vi "application.vi"() -> ()   [LabVIEW 2017, in "application.lvlib" / "application.lvclass"]
uses:
  application.lvclass
  application.lvclass/application.ctl
  <userlib>/NEVSTOP-Programming-Palette/Dialog & Interface/Fit VI window to Content_nevstop.vi
  <vilib>/Utility/config.llb/NI_LVConfig.lvlib
  <userlib>/NEVSTOP-Programming-Palette/Configuration/_OpenG Variant Configuration File/OpenG Variant Configuration File_nevstop.lvlib
panel:
  in  "Tab Control":enum32{"Main", "Settings"}(tab)
  out "version detected":string caption="File Path"
  in  "Settings":bool
  out "CMD":string caption="CMD Line"
  in  "file path":path=path "D:/Projects/Personal/Multi-LabVIEW-Selector/Multi-LabVIEW Selector.lvproj" caption="File Path"
  in  "LabVIEW List":string(combo)
  in  "OK":bool
  in  "Cancel":bool
  in  "Display Time(ms)":i32 min=0 max=10000 step=100
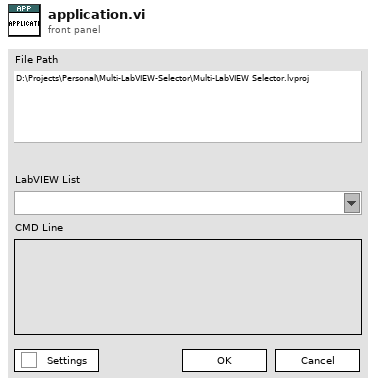
[diagram p1: front panel]
types:
  T1 = enum32{"invalid app kind", "Development System", "Run Time System", "Student Edition", "Embedded LabVIEW", "Evaluation", "Custom"}
  T2 = enum32{"Invalid", "Standard", "Closed", "Hidden", "Minimized", "Maximized"}
  T3 = cluster{"Core":cluster{"Current VI Reference":refnum<vi>, "Close Panel on Exit?":bool}, "RuntimeEngine":bool, "ConfigFilePath":path}
  T4 = cluster{"Current VI Reference":refnum<vi>, "Close Panel on Exit?":bool}
  T5 = typedef "NI_LVConfig.lvlib/Config Data RefNum.ctl" = refnum<k1>
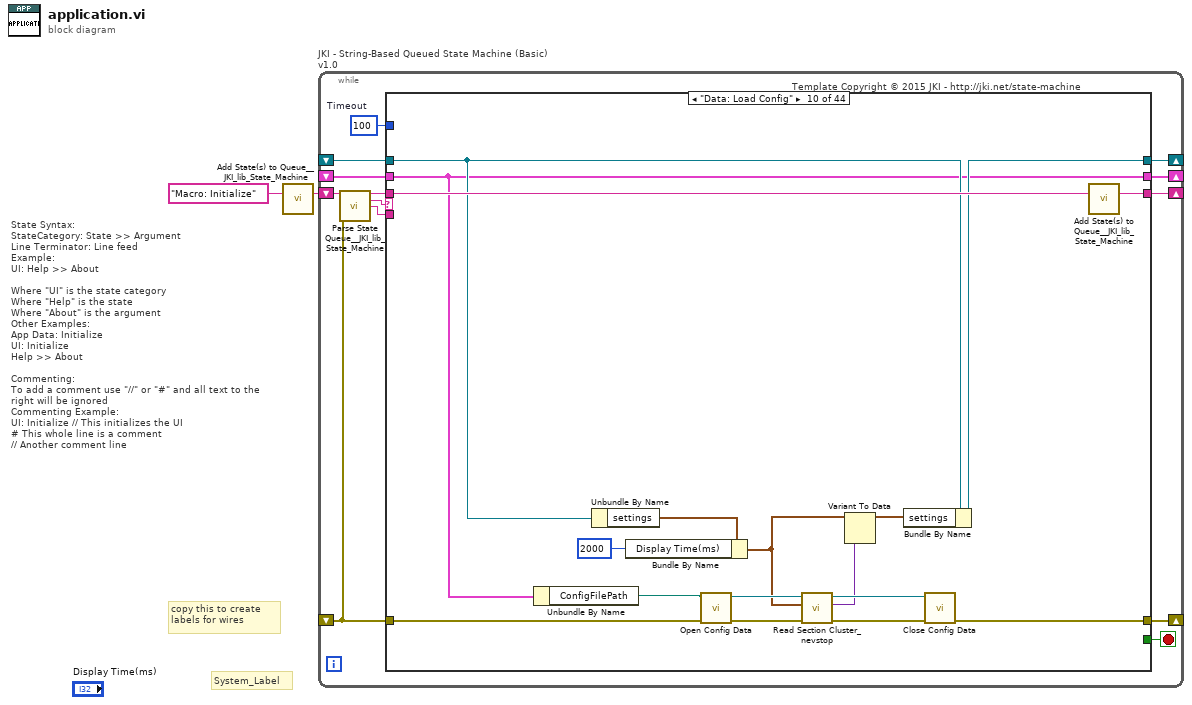
[diagram p0: block diagram]
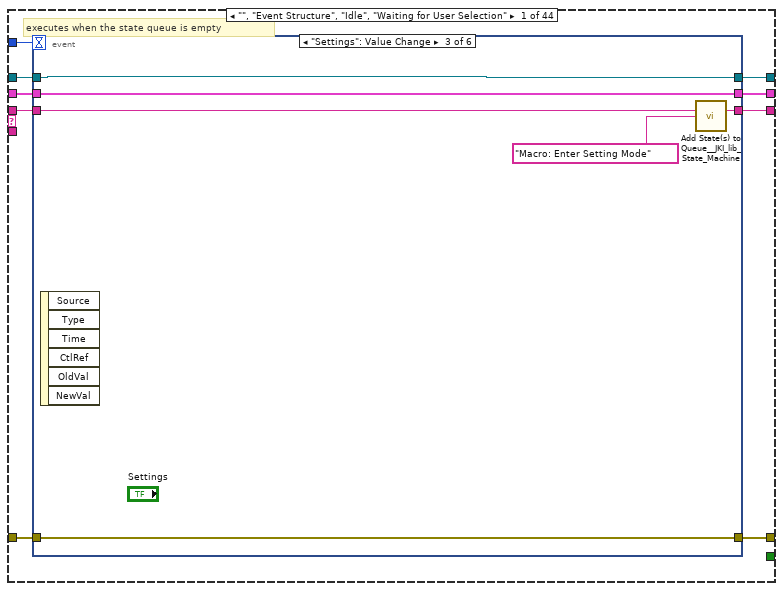
[diagram p2: hidden frame]
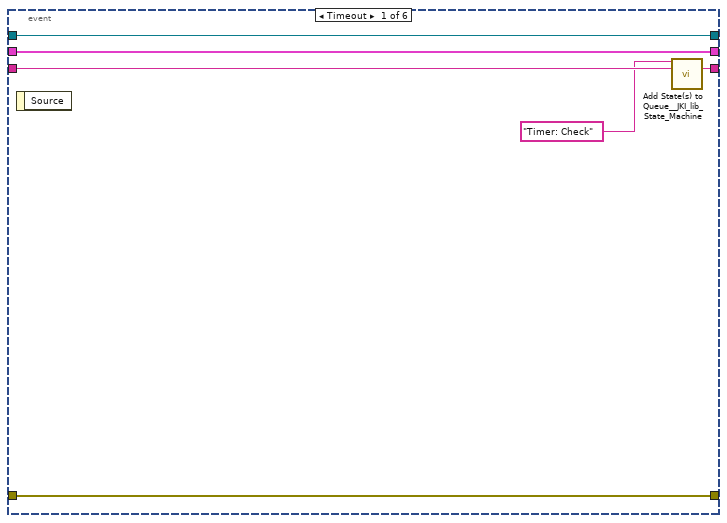
[diagram p3: hidden frame]
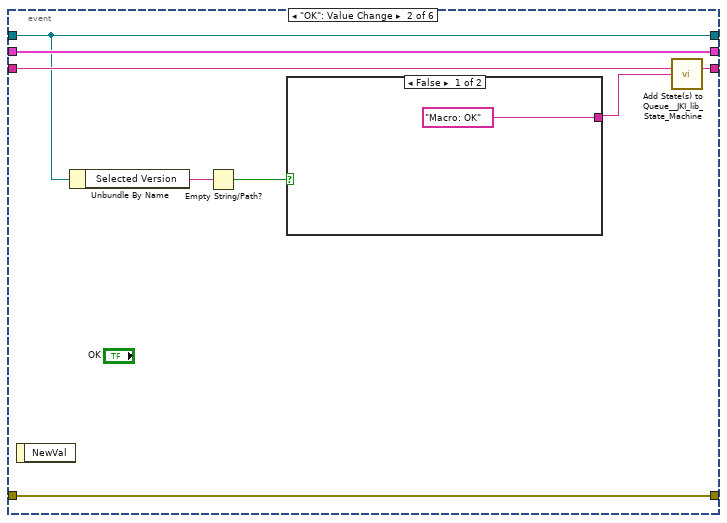
[diagram p4: hidden frame]
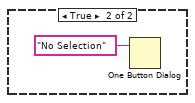
[diagram p5: hidden frame]
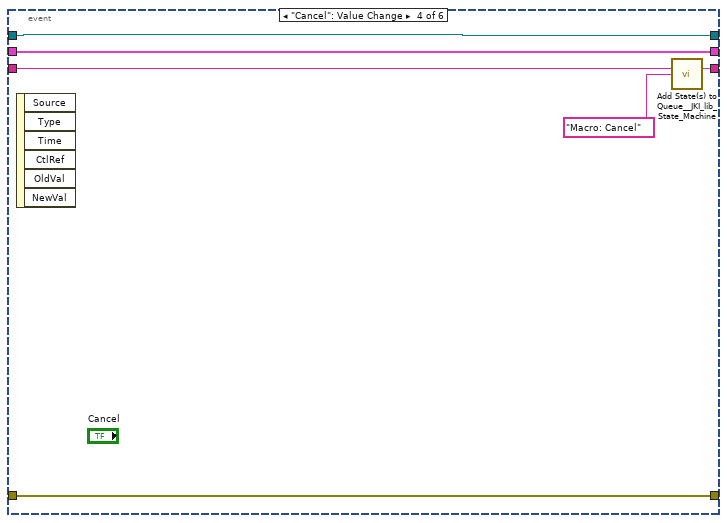
[diagram p6: hidden frame]
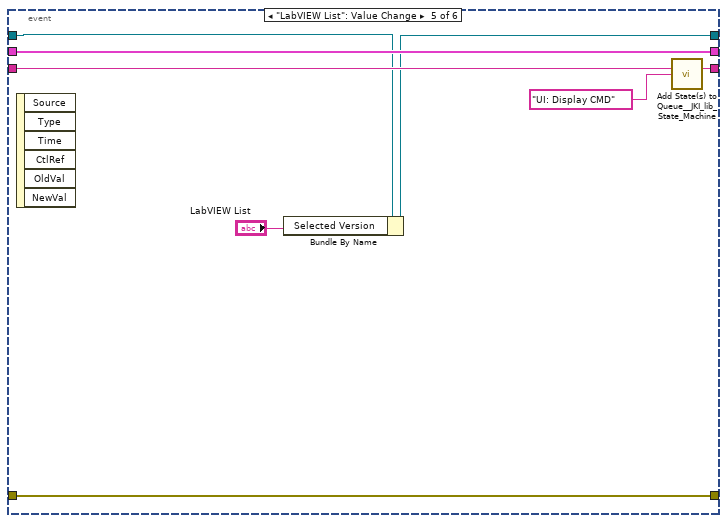
[diagram p7: hidden frame]
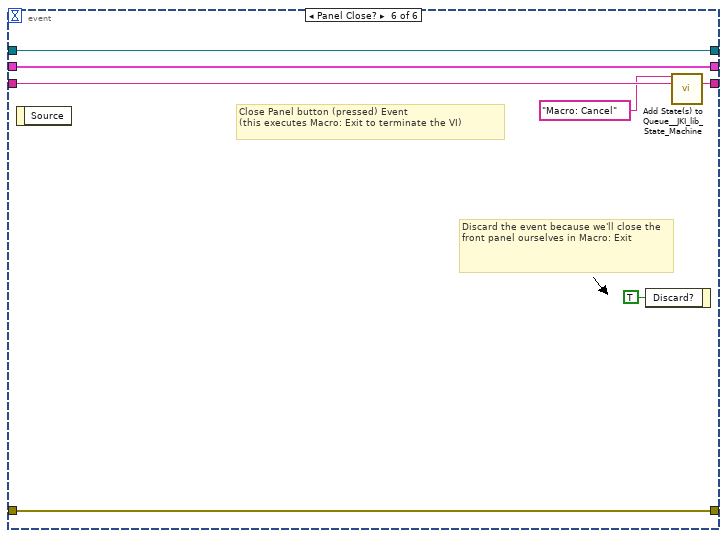
[diagram p8: hidden frame]
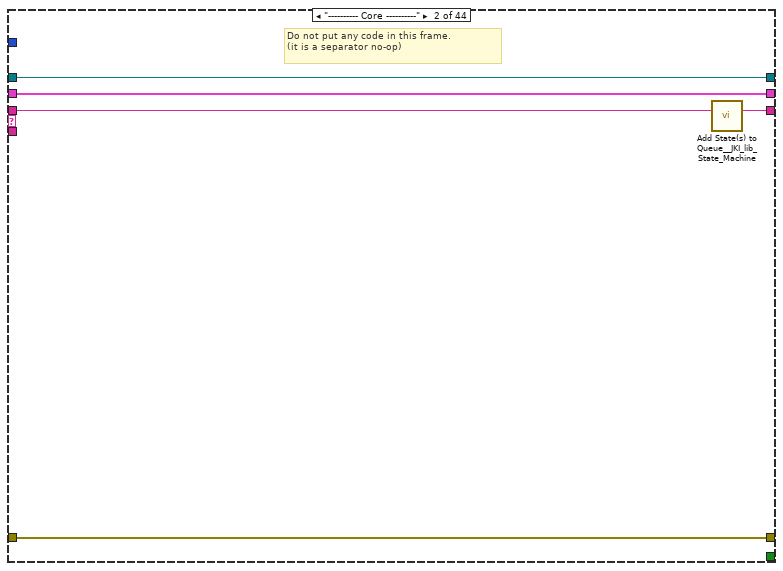
[diagram p9: hidden frame]
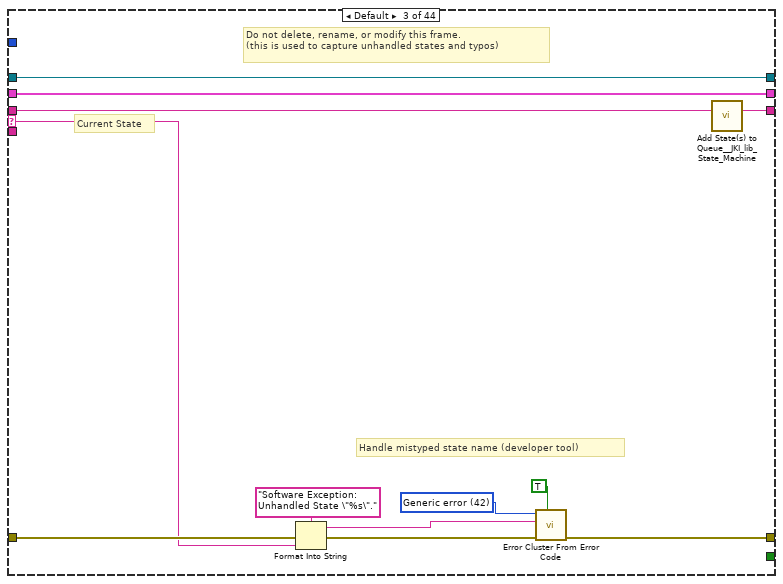
[diagram p10: hidden frame]
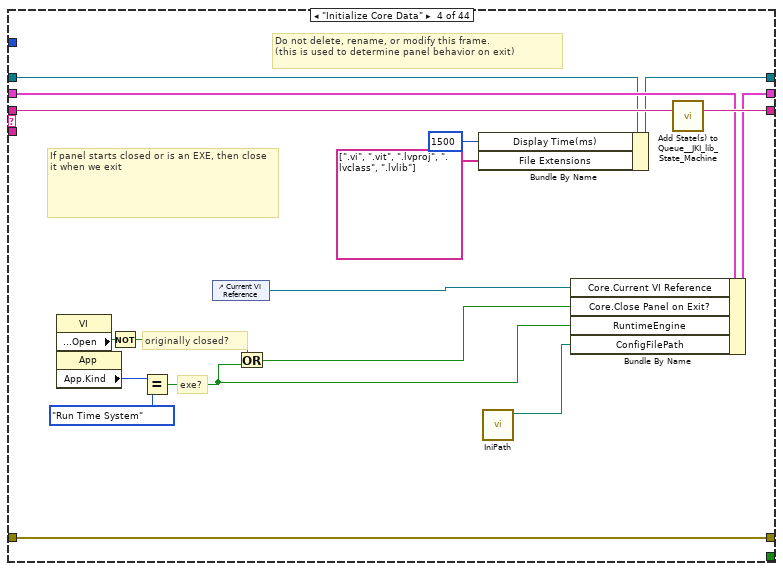
[diagram p11: hidden frame]
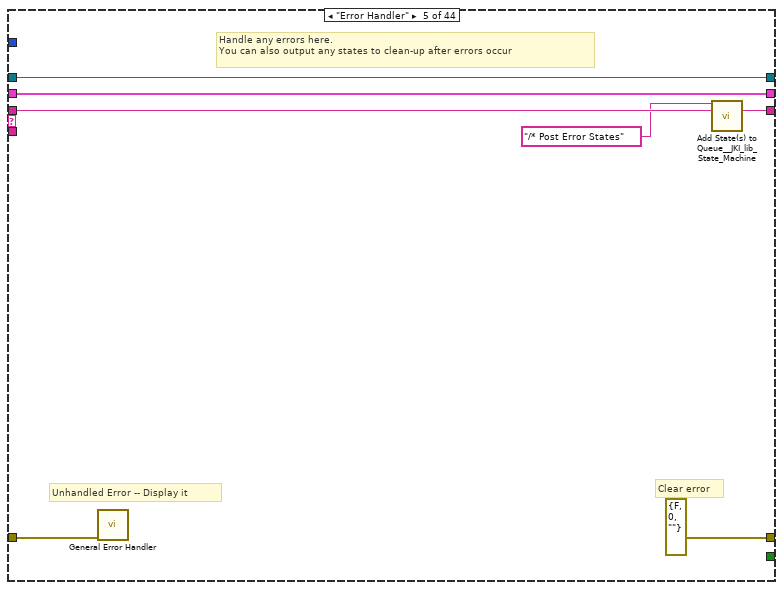
[diagram p12: hidden frame]
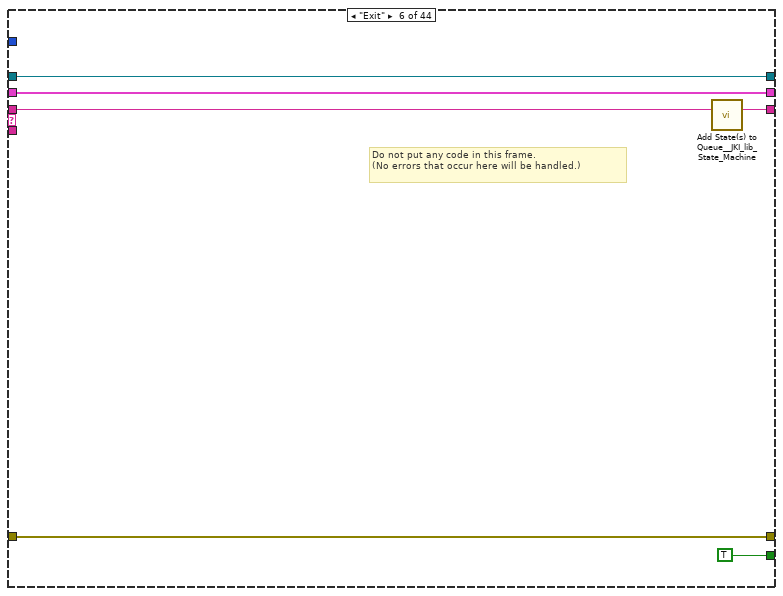
[diagram p13: hidden frame]
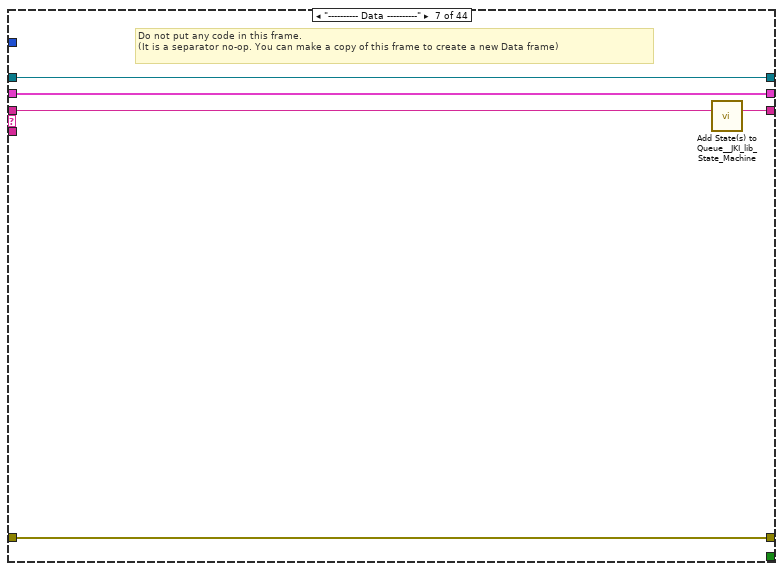
[diagram p14: hidden frame]
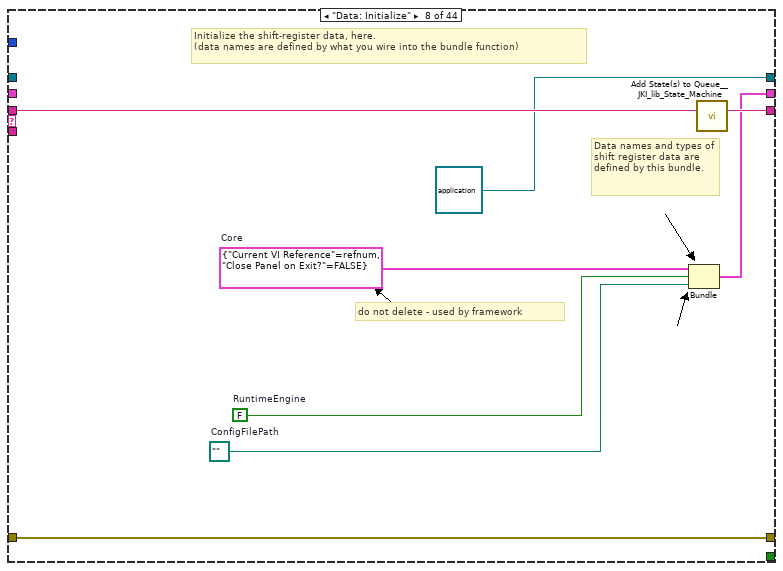
[diagram p15: hidden frame]
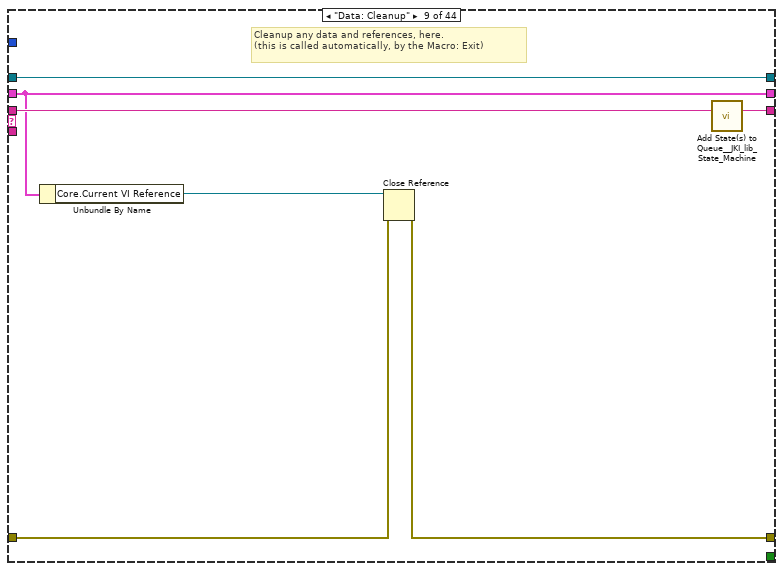
[diagram p16: hidden frame]
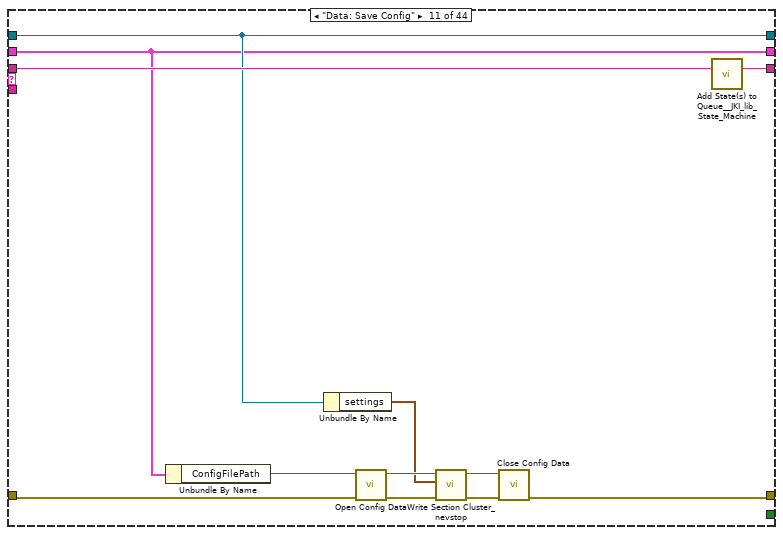
[diagram p17: hidden frame]
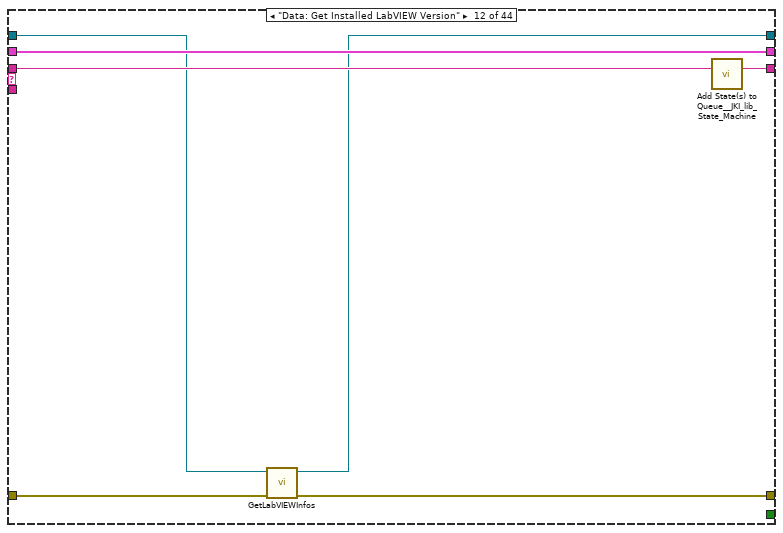
[diagram p18: hidden frame]
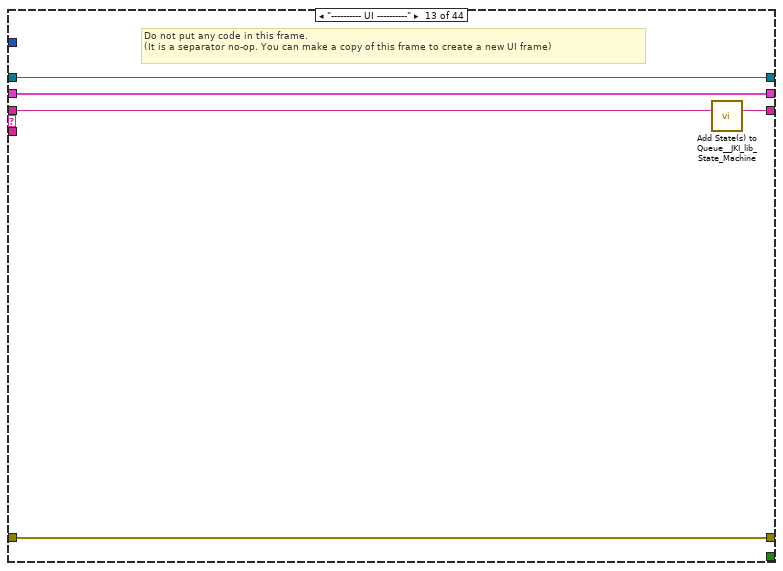
[diagram p19: hidden frame]
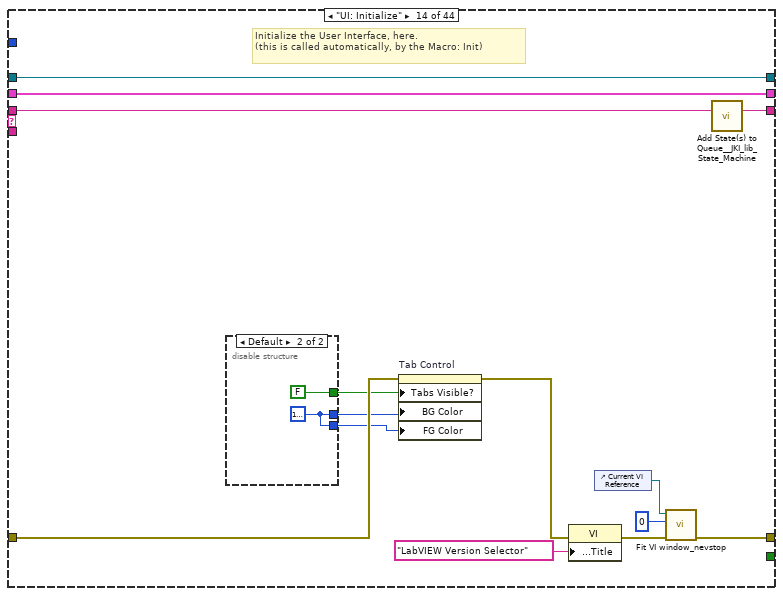
[diagram p20: hidden frame]
diagram:
  # "State Syntax:\nStateCategory: State >> Argument\nLine Terminator: Line feed\nExample:\nUI: Help >> About\n\nWhere \"UI\" is the state category\nWhere \"Help\" is the state\nWhere \"About\" is the argument\nOther Examples:\nApp Data: Initialize\nUI: Initialize\nHelp >> About\n\nCommenting:\nTo add a comment use \"//\" or \"#\" and all text to the right will be ignored\nCommenting Example:\nUI: Initialize // This initializes the UI\n# This whole line is a comment\n// Another comment line"
  # "copy this to create labels for wires"
  # "System_Label"
  n1 = call <vilib>:"Add State(s) to Queue__JKI_lib_State_Machine.vi"("State(s) in (\"\")"="Macro: Initialize") -> ("States Out"=w2:string)  [unwired: 14 in]
  n2 = while "JKI - String-Based Queued State Machine (Basic) v1.0" {
    shift-right: [w8] -> _
    shift-left: _ -> [w7]
    shift-right: [w11] -> _
    shift-left: _ -> [w5]
    shift-right: [w10] -> _
    shift-left: w2 -> [w12]
    shift-right: [w4] -> _
    shift-left: _ -> [w3]
    stop <- w9 stop-if-true
    w6 = 100  # Timeout
    # "Template Copyright © 2015 JKI - http://jki.net/state-machine"
    n3 = call <vilib>:"Parse State Queue__JKI_lib_State_Machine.vi"("State Queue"=w12, "Error In (no error)"=w5) -> ("Remaining States"=w14:string, "Current State"=w15:string, "Arguments"=w13:string)  [unwired: 11 in]
    n4 = case shown="\"Data: Load Config\"" w15 {
      selector: w15 -> [_ _ w74 _ _ _ _ _ _ _ _ _ _ _ _ _ _ _ _ _ _ _ _ _ _ _ _ _ _ _ _ _ _ _ _ _ _ _ _ _ _ _ _ _]
      tunnel: w14 -> [w24 w72 w78 w101 w108 w114 w119 w127 w134 w151 w163 w170 w175 w189 w200 w212 w243 w251 w260 w287 w294 w301 w307 w313 w319 w330 w336 w342 w347 w352 w365 w373 w380 w400 w406 w411 w420 w437 w454 w471 w483 w493 w512 w531]
      tunnel: w13 -> [_ _ _ _ _ _ _ _ _ _ _ _ _ _ w195 w206 _ _ _ _ w289 _ _ _ _ _ _ _ _ _ _ _ _ _ _ _ _ _ _ _ _ _ _ _]
      tunnel: w7 -> [w22 w69 w76 w93 w105 w112 w116 _ w129 w138 w152 w168 w172 w187 w198 w208 w241 w248 w257 w282 w291 w298 w304 w310 w316 w327 w333 w339 w344 w353 w362 w370 w377 w397 w403 w408 w416 w439 w456 w473 w485 w495 w514 w535]
      tunnel: [w21 w70 w80 w98 errorcluster {"status"=FALSE, "code"=0, "source"=""} ("error out") w111 w117 w124 w130 w143 w156 w166 w173 w185 w196 w209 w238 w249 w258 w285 w292 w299 w305 w311 w317 w328 w334 w340 w345 w350 w363 w371 w378 w398 w404 w409 w422 w435 w447 w464 w474 w491 w511 w532] -> w11
      tunnel: w5 -> [w20 w70 w79 w98 w104 w111 w117 w124 w131 w144 w155 w167 w173 w183 w197 w210 w239 w249 w258 w285 w292 w299 w305 w311 w317 w328 w334 w340 w345 w351 w363 w371 w378 w398 w404 w409 w423 w435 w448 w465 w475 w492 w511 w533]
      tunnel: [w23 w71 w77 w100 w107 w113 w118 w126 w133 w150 w162 w169 w174 w188 w199 w211 w242 w250 w259 w286 w293 w300 w306 w312 w318 w329 w335 w341 w346 w352 w364 w372 w379 w399 w405 w410 w421 w438 w455 w472 w484 w494 w513 w531] -> w10
      tunnel: [_ _ _ _ _ TRUE _ _ _ _ _ _ _ _ _ _ _ _ _ _ _ _ _ _ _ _ _ _ _ _ _ _ _ _ _ _ _ _ _ _ _ _ _ _] -> w9
      tunnel: [w19 w69 w76 w99 w105 w112 w116 w125 w129 w138 w152 w168 w172 w187 w198 w208 w241 w248 w257 w282 w291 w298 w304 w310 w316 w327 w333 w339 w344 w353 w362 w370 w377 w397 w403 w408 w416 w439 w456 w473 w485 w495 w514 w535] -> w8
      tunnel: w6 -> [w18 _ _ _ _ _ _ _ _ _ _ _ _ _ _ _ _ _ _ _ _ _ _ _ _ _ _ _ _ _ _ _ _ _ _ _ _ _ _ _ _ _ _ _]
      tunnel: [w16 w68 w73 w89 w102 w109 w115 refnum<class "application.lvclass"> refnum ("application.lvclass") w128 w142 w154 w164 w171 w186 w194 w205 w236 w245 w256 w284 w290 w297 w302 w308 w314 w320 w332 w338 w343 w354 w361 w368 w375 w395 w402 w407 w419 w436 w449 w466 w476 w490 w506 w534] -> w4
      tunnel: w3 -> [w17 w68 w73 w90 w102 w109 w115 _ w128 w149 w154 w165 w171 w186 w194 w205 w237 w245 w256 w284 w290 w297 w302 w308 w314 w320 w332 w338 w343 w354 w361 w369 w376 w395 w402 w407 w424 w436 w450 w467 w476 w490 w507 w534]
      frame "", "Event Structure", "Idle", "Waiting for User Selection" {
        # "executes when the state queue is empty"
        n5 = event shown="[2] \"Settings\": Value Change" {
          selector: _ -> [_ _ _ _ _ _]
          dyn-events: _ -> [_ _ _ _ _ _]
          timeout: w18 -> [_ _ _ _ _ _]
          tunnel: w24 -> [w30 w38 w46 w52 w60 w67]
          tunnel: [w29 w37 w45 w51 w59 w66] -> w23
          tunnel: w22 -> [w27 w36 w43 w49 w57 w64]
          tunnel: [w28 w35 w44 w50 w58 w65] -> w21
          tunnel: w20 -> [w28 w35 w44 w50 w58 w65]
          tunnel: [w27 w36 w43 w49 w57 w64] -> w19
          tunnel: w17 -> [w26 w34 w42 w48 w56 w61]
          tunnel: [w26 w34 w42 w48 w54 w61] -> w16
          event Timeout {
            n6 = event-data() -> ()  [unwired: 1 in, 1 out]
            n7 = call <vilib>:"Add State(s) to Queue__JKI_lib_State_Machine.vi"("State(s) in Front (\"\")"="Timer: Check" ("State(s) in Front (\"\")"), "State(s) in (\"\")"=w30) -> ("States Out"=w29:string)  [unwired: 13 in]
          }
          event "OK": Value Change {
            n8 = event-data() -> ()  [unwired: 1 in, 1 out]
            n9 = Unbundle By Name(w34) -> ("Selected Version"=w33:string)
            n10 = Empty String/Path?(string/path=w33) -> (empty?=w32:bool)
            n11 = case shown="False" w32 {
              tunnel: ["Macro: OK" ("State(s) at Back (\"\")") _] -> w31
              frame False {
              }
              frame True {
                n12 = One Button Dialog(message="No Selection") -> ()  [unwired: 1 in, 1 out]
              }
            }
            n13 = call <vilib>:"Add State(s) to Queue__JKI_lib_State_Machine.vi"("State(s) in (\"\")"=w38, "State(s) at Back (\"\")"=w31) -> ("States Out"=w37:string)  [unwired: 13 in]
          }
          event "Settings": Value Change {
            n14 = event-data() -> ()  [unwired: 1 in, 6 out]
            n15 = call <vilib>:"Add State(s) to Queue__JKI_lib_State_Machine.vi"("State(s) in (\"\")"=w46, "State(s) at Back (\"\")"="Macro: Enter Setting Mode" ("State(s) at Back (\"\")")) -> ("States Out"=w45:string)  [unwired: 13 in]
          }
          event "Cancel": Value Change {
            n16 = event-data() -> ()  [unwired: 1 in, 6 out]
            n17 = call <vilib>:"Add State(s) to Queue__JKI_lib_State_Machine.vi"("State(s) in (\"\")"=w52, "State(s) at Back (\"\")"="Macro: Cancel" ("State(s) at Back (\"\")")) -> ("States Out"=w51:string)  [unwired: 13 in]
          }
          event "LabVIEW List": Value Change {
            n18 = event-data() -> ()  [unwired: 1 in, 6 out]
            n19 = Bundle By Name(cluster=w56, "Selected Version"="LabVIEW List") -> (w54:refnum<class "application.lvclass">)
            n20 = call <vilib>:"Add State(s) to Queue__JKI_lib_State_Machine.vi"("State(s) in (\"\")"=w60, "State(s) at Back (\"\")"="UI: Display CMD" ("State(s) at Back (\"\")")) -> ("States Out"=w59:string)  [unwired: 13 in]
          }
          event Panel Close? {
            # "Discard the event because we'll close the front panel ourselves in Macro: Exit"
            # "Close Panel button (pressed) Event\n(this executes Macro: Exit to terminate the VI)"
            n21 = event-data() -> ()  [unwired: 1 in, 1 out]
            n22 = event-data("Discard?"=TRUE) -> ()  [unwired: 1 in, 1 out]
            n23 = call <vilib>:"Add State(s) to Queue__JKI_lib_State_Machine.vi"("State(s) in Front (\"\")"="Macro: Cancel", "State(s) in (\"\")"=w67) -> ("States Out"=w66:string)  [unwired: 13 in]
          }
        }
      }
      frame "---------- Core ----------" {
        # "Do not put any code in this frame.\n(it is a separator no-op)"
        n24 = call <vilib>:"Add State(s) to Queue__JKI_lib_State_Machine.vi"("State(s) in (\"\")"=w72) -> ("States Out"=w71:string)  [unwired: 14 in]
      }
      frame Default {
        w83 = 42 items=["No error", "Argument error", "Memory is full", "Out of zone", "End of file", "File already open", "Generic file I/O error", "File not found", "File permission error", "Disk is full", "Duplicate path", "Too many files open", "System feature not enabled", "Resource file not found", "Cannot add resource", "Resource not found", "Image not found", "Image memory error", "Pen does not exist", "Config type invalid", "Config token not found", "Config parse error", "Config memory error", "Bad external code format", "Bad external code offset", "External code not present", "Null window", "Destroy window error", "Null menu", "Print aborted", "Bad print record", "Print driver error", "Windows error during printing", "Memory error during printing", "Print dialog error", "Generic print error", "Invalid device refnum", "Device not found", "Device parameter error", "Device unit error", "Cannot open device", "Device call aborted", "Generic error", "Cancelled by user", "Object ID too low", "Object ID too high", "Object not in heap", "Unknown heap", "Unknown object (invalid DefProc)", "Unknown object (DefProc not in table)", "Message out of range", "Invalid (null) method", "Unknown message", "Manager call not supported", "Bad address", "Network operation in progress", "Network operation timed out", "Connection is busy", "Network attribute not supported", "Network error", "Address in use", "System out of memory", "Connection aborted", "Connection refused", "Not connected", "Already connected", "Connection closed", "Initialization error (interapplication manager)", "Bad occurrence", "Wait on unbound occurrence handler", "Occurrence queue overflow", "Datalog type conflict", "Unused", "Unrecognized type (interapplication manager)", "Memory corrupt", "Failed to make temporary DLL", "Old CIN version", "Drag socket not found", "Failed to load drop-object", "Failed to register OLE object", "Failed to release OLE object", "Format specifier type mismatch", "Unknown format specifier", "Too few format specifiers", "Too many format specifiers", "Scan failed", "Newer CIN version", "Error converting to variant", "Runtime menu error", "Password tampered", "Variant attribute not found", "Incompatible variant data type", "Event data is not available", "Event Store is not present", "Occurrence is not found", "Event Queue is not created", "Event info is not available", "Refnum passed is NULL", "Error retrieving Class GUID", "Error retrieving CoClass GUID", "Error retrieving TypeLib GUID.", "Bad built application magic bytes.", "Specific driver is different from the specific driver associated with the Logical Name.", "There is no session opened to the class driver.", "Max Error", "MAX - Error with config objects", "MAX - Error loading configuration", "MAX - Group not supported"]
        # "Current State"
        # "Do not delete, rename, or modify this frame.\n(this is used to capture unhandled states and typos)"
        # "Handle mistyped state name (developer tool)"
        n25 = Format Into String(format string="Software Exception: Unhandled State \"%s\"." ("message"), error in=w79, w74) -> (resulting string=w82:string, error out=w81:errorcluster)  [unwired: 1 in]
        n26 = call <vilib>:"Error Cluster From Error Code.vi"("show call chain? (False)"=TRUE, "error in (no error)"=w81, "error message (\"\")"=w82, "error code (0)"=w83) -> ("error out"=w80:errorcluster)  [unwired: 5 in]
        n27 = call <vilib>:"Add State(s) to Queue__JKI_lib_State_Machine.vi"("State(s) in (\"\")"=w78) -> ("States Out"=w77:string)  [unwired: 14 in]
      }
      frame "Initialize Core Data" {
        # "Do not delete, rename, or modify this frame.\n(this is used to determine panel behavior on exit)"
        # "originally closed?"
        # "exe?"
        # "If panel starts closed or is an EXE, then close it when we exit"
        n28 = property class="VI"() -> ("Front Panel.Open"=w97:bool)  [unwired: 2 in, 2 out]
        n29 = property class="App"() -> ("App.Kind"=w96:T1)  [unwired: 2 in, 2 out]
        n30 = Not(x=w97) -> (.not. x?=w94:bool)
        n31 = Equal?(x=w96, y=T1."Run Time System" ("Application:Kind")) -> (x = y?=w85:bool)
        n32 = control-ref of="Current VI Reference"() -> (w91:refnum<vi>)
        n33 = Or(x=w94, y=w85) -> (x .or. y?=w92:bool)
        n34 = Bundle By Name(cluster=w90, "Display Time(ms)"=1500 ("settings.Display Time(ms)"), "File Extensions"=string[] [".vi", ".vit", ".lvproj", ".lvclass", ".lvlib"]) -> (w89:refnum<class "application.lvclass">)
        n35 = call "IniPath.vi"() -> ("INI Path"=w86:path)  [unwired: 11 in]
        n36 = Bundle By Name(cluster=w93, "Core.Current VI Reference"=w91, "Core.Close Panel on Exit?"=w92, "RuntimeEngine"=w85, "ConfigFilePath"=w86) -> (w99:T3)
        n37 = call <vilib>:"Add State(s) to Queue__JKI_lib_State_Machine.vi"("State(s) in (\"\")"=w101) -> ("States Out"=w100:string)  [unwired: 14 in]
      }
      frame "Error Handler" {
        # "Unhandled Error -- Display it"
        # "Handle any errors here.\nYou can also output any states to clean-up after errors occur"
        # "Clear error"
        n38 = call <vilib>:"General Error Handler.vi"("error in (no error)"=w104) -> ()  [unwired: 10 in, 5 out]
        n39 = call <vilib>:"Add State(s) to Queue__JKI_lib_State_Machine.vi"("State(s) in Front (\"\")"="/* Post Error States", "State(s) in (\"\")"=w108) -> ("States Out"=w107:string)  [unwired: 13 in]
      }
      frame "Exit" {
        # "Do not put any code in this frame.\n(No errors that occur here will be handled.)"
        n40 = call <vilib>:"Add State(s) to Queue__JKI_lib_State_Machine.vi"("State(s) in (\"\")"=w114) -> ("States Out"=w113:string)  [unwired: 14 in]
      }
      frame "---------- Data ----------" {
        # "Do not put any code in this frame.\n(It is a separator no-op. You can make a copy of this frame to create a new Data frame)"
        n41 = call <vilib>:"Add State(s) to Queue__JKI_lib_State_Machine.vi"("State(s) in (\"\")"=w119) -> ("States Out"=w118:string)  [unwired: 14 in]
      }
      frame "Data: Initialize" {
        w121 = T4 {"Current VI Reference"=refnum, "Close Panel on Exit?"=FALSE}  # Core
        w123 = FALSE  # RuntimeEngine
        w122 = path ""  # ConfigFilePath
        # "do not delete - used by framework"
        # "Data names and types of shift register data are defined by this bundle."
        # "Initialize the shift-register data, here.\n(data names are defined by what you wire into the bundle function)"
        n42 = Bundle("Core"=w121, "RuntimeEngine"=w123, "ConfigFilePath"=w122) -> (w125:T3)  [unwired: 1 in]
        n43 = call <vilib>:"Add State(s) to Queue__JKI_lib_State_Machine.vi"("State(s) in (\"\")"=w127) -> ("States Out"=w126:string)  [unwired: 14 in]
      }
      frame "Data: Cleanup" {
        # "Cleanup any data and references, here.\n(this is called automatically, by the Macro: Exit)"
        n44 = Unbundle By Name(w129) -> ("Core.Current VI Reference"=w132:refnum<vi>)
        n45 = Close Reference(reference=w132, error in (no error)=w131) -> (error out=w130:errorcluster)
        n46 = call <vilib>:"Add State(s) to Queue__JKI_lib_State_Machine.vi"("State(s) in (\"\")"=w134) -> ("States Out"=w133:string)  [unwired: 14 in]
      }
      frame "Data: Load Config" {
        n47 = Unbundle By Name(w138) -> ("ConfigFilePath"=w137:path)
        n48 = Unbundle By Name(w149) -> ("settings"=w139:cluster{"Display Time(ms)":i32})
        n49 = Bundle By Name(cluster=w139, "Display Time(ms)"=2000) -> (w136:cluster{"Display Time(ms)":i32})
        n50 = call <vilib>:"Open Config Data.vi"("error in (no error)"=w144, "configuration file path"=w137) -> ("error out"=w147:errorcluster, "refnum"=w148:T5)  [unwired: 7 in, 1 out]
        n51 = call <userlib>:"Read Section Cluster_nevstop.vi"("error in (no error)"=w147, "Section Formatted Cluster Type"=w136, "refnum"=w148) -> ("error out"=w145:errorcluster, "Section Formatted Cluster"=w140:variant, "dup refnum"=w146:T5)  [unwired: 4 in, 2 out]
        n52 = Variant To Data(type=w136, Variant=w140) -> (data=w141:cluster{"Display Time(ms)":i32})  [unwired: 1 in, 1 out]
        n53 = Bundle By Name(cluster=w149, "settings"=w141) -> (w142:refnum<class "application.lvclass">)
        n54 = call <vilib>:"Close Config Data.vi"("error in (no error)"=w145, "refnum"=w146) -> ("error out"=w143:errorcluster)  [unwired: 8 in, 1 out]
        n55 = call <vilib>:"Add State(s) to Queue__JKI_lib_State_Machine.vi"("State(s) in (\"\")"=w151) -> ("States Out"=w150:string)  [unwired: 14 in]
      }
      frame "Data: Save Config" {
        n56 = Unbundle By Name(w152) -> ("ConfigFilePath"=w153:path)
        n57 = Unbundle By Name(w154) -> ("settings"=w157:cluster{"Display Time(ms)":i32})
        n58 = call <vilib>:"Open Config Data.vi"("error in (no error)"=w155, "configuration file path"=w153) -> ("error out"=w160:errorcluster, "refnum"=w161:T5)  [unwired: 7 in, 1 out]
        n59 = call <userlib>:"Write Section Cluster_nevstop.vi"("error in (no error)"=w160, "Section Formatted Cluster"=w157, "refnum"=w161) -> ("error out"=w158:errorcluster, "dup refnum"=w159:T5)  [unwired: 7 in]
        n60 = call <vilib>:"Close Config Data.vi"("error in (no error)"=w158, "refnum"=w159) -> ("error out"=w156:errorcluster)  [unwired: 8 in, 1 out]
        n61 = call <vilib>:"Add State(s) to Queue__JKI_lib_State_Machine.vi"("State(s) in (\"\")"=w163) -> ("States Out"=w162:string)  [unwired: 14 in]
      }
      frame "Data: Get Installed LabVIEW Version" {
        n62 = call "GetLabVIEWInfos.vi"("error in (no error)"=w167, "application.lvclass"=w165) -> ("error out"=w166:errorcluster, "application.lvclass (dup)"=w164:refnum<class "application.lvclass">)  [unwired: 8 in]
        n63 = call <vilib>:"Add State(s) to Queue__JKI_lib_State_Machine.vi"("State(s) in (\"\")"=w170) -> ("States Out"=w169:string)  [unwired: 14 in]
      }
      frame "---------- UI ----------" {
        # "Do not put any code in this frame.\n(It is a separator no-op. You can make a copy of this frame to create a new UI frame)"
        n64 = call <vilib>:"Add State(s) to Queue__JKI_lib_State_Machine.vi"("State(s) in (\"\")"=w175) -> ("States Out"=w174:string)  [unwired: 14 in]
      }
      frame "UI: Initialize" {
        # "Initialize the User Interface, here.\n(this is called automatically, by the Macro: Init)"
        n65 = disable-structure shown="Default" {
          disable-tunnel: [FALSE ("Tabs Visible?") FALSE ("Tabs Visible?")] -> w182
          disable-tunnel: [w190 w192] -> w181
          disable-tunnel: [w190 w192] -> w180
          frame condition #0 {
            w190 = u32 16777216
          }
          frame condition #1 (active) {
            w192 = u32 16777216
          }
        }
        n66 = property on="Tab Control" class="TabCtl (strict)"(error in=w183, "Tabs Visible?"=w182, "BG Color"=w181, "FG Color"=w180) -> (error out=w178:errorcluster)  [unwired: 1 in, 1 out]
        n67 = property class="VI"(error in=w178, "Front Panel.Title"="LabVIEW Version Selector" ("Front Panel Window:Title")) -> (error out=w177:errorcluster)  [unwired: 1 in, 1 out]
        n68 = control-ref of="Current VI Reference"() -> (w176:refnum<vi>)
        n69 = call-poly <userlib>:"Fit VI window_nevstop.vi"("error in (no error)"=w177, "border spacing (2 px)"=0, "VI Ref (calling VI)"=w176) -> ("error out"=w185:errorcluster)  [unwired: 3 in, 1 out]
        n70 = call <vilib>:"Add State(s) to Queue__JKI_lib_State_Machine.vi"("State(s) in (\"\")"=w189) -> ("States Out"=w188:string)  [unwired: 14 in]
      }
      frame "UI: Cursor Set" {
        # "Argument"
        # "Set and Unset Cursor Busy.\n(Usage: \"UI: Cursor Set >> Busy|Idle\")"
        n71 = case shown="\"Idle\", Default" w195 {
          tunnel: w197 -> [w202 w204]
          tunnel: [w201 w203] -> w196
          frame "Idle", Default {
            n72 = call <vilib>:"Unset Busy.vi"("error in (no error)"=w202) -> ("error out"=w201:errorcluster)  [unwired: 10 in]
          }
          frame "Busy" {
            n73 = call <vilib>:"Set Busy.vi"("error in (no error)"=w204) -> ("error out"=w203:errorcluster)  [unwired: 9 in, 1 out]
          }
        }
        n74 = call <vilib>:"Add State(s) to Queue__JKI_lib_State_Machine.vi"("State(s) in (\"\")"=w200) -> ("States Out"=w199:string)  [unwired: 14 in]
      }
      frame "UI: Front Panel State" {
        # "Argument"
        # "Set Front Panel Open or Closed\n(Usage: \"UI: Front Panel State >> Open|Close\")"
        n75 = Unbundle By Name(w208) -> ("Core.Current VI Reference"=w207:refnum<vi>)
        n76 = case shown="\"Open\", Default" w206 {
          tunnel: w210 -> [w216 w229]
          tunnel: [w218 w230] -> w209
          tunnel: w207 -> [w217 w227]
          frame "Open", Default {
            n77 = property class="VI"(reference=w217, error in=w216) -> (reference out=w214:refnum<vi>, error out=w215:errorcluster, "Front Panel.Open"=w213:bool)
            n78 = case shown="False" w213 {
              tunnel: [w221 w224] -> w218
              tunnel: w215 -> [w220 w224]
              tunnel: w214 -> [w219 _]
              frame False {
                n79 = invoke class="VI" method="FP.Open"(reference=w219, error in=w220, "Activate"=TRUE, "State"=T2."Standard") -> (error out=w221:errorcluster)  [unwired: 1 in, 4 out]
              }
              frame True {
              }
            }
          }
          frame "Close" {
            n80 = property class="VI"(reference=w227, error in=w229) -> (reference out=w226:refnum<vi>, error out=w228:errorcluster, "Front Panel.Open"=w225:bool)
            n81 = case shown="True" w225 {
              tunnel: [w231 w234] -> w230
              tunnel: w228 -> [w231 w233]
              tunnel: w226 -> [_ w232]
              frame False {
              }
              frame True {
                n82 = invoke class="VI" method="FP.Close"(reference=w232, error in=w233) -> (error out=w234:errorcluster)  [unwired: 1 in, 2 out]
              }
            }
          }
        }
        n83 = call <vilib>:"Add State(s) to Queue__JKI_lib_State_Machine.vi"("State(s) in (\"\")"=w212) -> ("States Out"=w211:string)  [unwired: 14 in]
      }
      frame "UI: Display CMD" {
        n84 = call "GetCMDLine.vi"("error in (no error)"=w239, "application in"=w237) -> ("error out"=w238:errorcluster, "application out"=w236:refnum<class "application.lvclass">)  [unwired: 8 in]
        n85 = Unbundle By Name(w236) -> ("File Path"=w235:path, "CMD line"=→"CMD":string)
        n86 = local write "file path"(w235) -> ()
        n87 = call <vilib>:"Add State(s) to Queue__JKI_lib_State_Machine.vi"("State(s) in (\"\")"=w243) -> ("States Out"=w242:string)  [unwired: 14 in]
      }
      frame "UI: Display LabVIEW Information" {
        n88 = Unbundle By Name(w245) -> ("Version List"=w247:string[], "Selected Version"=w246:string)
        n89 = control-ref of="LabVIEW List"() -> (w244:refnum<vi>)
        n90 = property on="Property Node" class="CmbBox"(reference=w244, "Strings[]"=w247, "Value"=w246) -> ()  [unwired: 1 in, 2 out]
        n91 = call <vilib>:"Add State(s) to Queue__JKI_lib_State_Machine.vi"("State(s) in (\"\")"=w251) -> ("States Out"=w250:string)  [unwired: 14 in]
      }
      frame "UI: Display LV Version in Source file" {
        n92 = Unbundle By Name(w256) -> ("File Path"=w255:path)
        n93 = call <vilib>:"Check if File or Folder Exists.vi"("path"=w255) -> ("error out"=w252:errorcluster, "file or folder exists?"=w253:bool, "dup path"=w254:path)  [unwired: 8 in]
        n94 = case shown="True" w253 {
          tunnel: w254 -> [_ w263]
          tunnel: w252 -> [_ w262]
          frame False {
          }
          frame True {
            n95 = call <vilib>:"Get File Extension.vi"("error in (no error)"=w262, "file"=w263) -> ("lowercase file extension"=w265:string, "dup file"=w266:path)  [unwired: 5 in, 3 out]
            n96 = case shown="\"ctl\", \"ctt\", \"vi\", \"vim\", \"vit\"" w265 {
              selector: w265 -> [_ w270 w280]
              tunnel: w266 -> [_ w273 w277]
              tunnel: [_ w271 w281] -> w264
              tunnel: "File Extension: " ("string") -> [_ w267 w274]
              frame "False", Default {
              }
              frame "lvclass", "lvlib", "lvproj" {
                n97 = call "_lvVersion - xml.vi"("Path"=w273) -> ("text"=w272:string)  [unwired: 8 in, 2 out]
                n98 = Concatenate Strings(w267, w270, "   " ("string"), "LabVIEW Version:" ("string"), w272) -> (w271:string)
              }
              frame "ctl", "ctt", "vi", "vim", "vit" {
                n99 = invoke class="App" method="Get VI Version"("path"=w277) -> ("GetVIVers"=w275:string)  [unwired: 4 in, 4 out]
                n100 = Format Into String(w275) -> (resulting string=w276:string)  [unwired: 3 in, 1 out]
                n101 = Concatenate Strings(w274, w280, "  " ("string"), "LabVIEW Version:" ("string"), w276) -> (w281:string)
              }
            }
            "version detected" <- w264
          }
        }
        n102 = call <vilib>:"Add State(s) to Queue__JKI_lib_State_Machine.vi"("State(s) in (\"\")"=w260) -> ("States Out"=w259:string)  [unwired: 14 in]
      }
      frame "UI: Display Settings" {
        n103 = Unbundle By Name(w284) -> ("Display Time(ms)"=w283:i32)
        n104 = local write "Display Time(ms)"(w283) -> ()
        n105 = call <vilib>:"Add State(s) to Queue__JKI_lib_State_Machine.vi"("State(s) in (\"\")"=w287) -> ("States Out"=w286:string)  [unwired: 14 in]
      }
      frame "UI: Switch Page" {
        n106 = case shown="\"Settings\"" w289 {
          tunnel: [enum32{"Main", "Settings"}."Settings" ("Tab Control") enum32{"Main", "Settings"}."Main" ("Tab Control")] -> w288
          frame "Settings" {
          }
          frame Default {
          }
        }
        n107 = local write "Tab Control"(w288) -> ()
        n108 = call <vilib>:"Add State(s) to Queue__JKI_lib_State_Machine.vi"("State(s) in (\"\")"=w294) -> ("States Out"=w293:string)  [unwired: 14 in]
      }
      frame "---------- Macro ----------" {
        # "Do not put any code in this frame.\n(It is a separator no-op. You can make a copy of this frame to create a new Macro frame)"
        n109 = call <vilib>:"Add State(s) to Queue__JKI_lib_State_Machine.vi"("State(s) in (\"\")"=w301) -> ("States Out"=w300:string)  [unwired: 14 in]
      }
      frame "Macro: Initialize" {
        # "Initialization Macro\n(This is called once, when the VI starts)"
        n110 = call <vilib>:"Add State(s) to Queue__JKI_lib_State_Machine.vi"("State(s) in Front (\"\")"="Data: Initialize\nInitialize Core Data\nData: Load Config\nData: Get Installed LabVIEW Version\nUI: Initialize\nUI: Front Panel State >> Open\nRegister Exts\nGet Opened File Name\nUI: Display LV Version in Source file\nUI: Display LabVIEW Information\nUI: Display Settings\nUI: Display CMD", "State(s) in (\"\")"=w307) -> ("States Out"=w306:string)  [unwired: 13 in]
      }
      frame "Macro: OK" {
        # "Initialization Macro\n(This is called once, when the VI starts)"
        n111 = call <vilib>:"Add State(s) to Queue__JKI_lib_State_Machine.vi"("State(s) in Front (\"\")"="Update Symbol\nExcute CMD\nMacro: Exit", "State(s) in (\"\")"=w313) -> ("States Out"=w312:string)  [unwired: 13 in]
      }
      frame "Macro: Cancel" {
        # "Initialization Macro\n(This is called once, when the VI starts)"
        n112 = call <vilib>:"Add State(s) to Queue__JKI_lib_State_Machine.vi"("State(s) in Front (\"\")"="Macro: Exit", "State(s) in (\"\")"=w319) -> ("States Out"=w318:string)  [unwired: 13 in]
      }
      frame "Macro: Exit" {
        # "Exit Macro\n(This is called once, when the VI exits)"
        n113 = Unbundle By Name(w327) -> ("Core.Close Panel on Exit?"=w326:bool)
        n114 = Select(t="UI: Front Panel State >> Close", s=w326, f="") -> (s? t:f=w323:string)
        n115 = call <vilib>:"Add State(s) to Queue__JKI_lib_State_Machine.vi"("State(s) in (\"\")"=w323, "State(s) at Back (\"\")"="Data: Save Config\nData: Cleanup\nExit") -> ("States Out"=w321:string)  [unwired: 13 in]
        n116 = call <vilib>:"Add State(s) to Queue__JKI_lib_State_Machine.vi"("State(s) in Front (\"\")"=w321, "State(s) in (\"\")"=w330) -> ("States Out"=w329:string)  [unwired: 13 in]
      }
      frame "Macro: Enter Setting Mode" {
        n117 = call <vilib>:"Add State(s) to Queue__JKI_lib_State_Machine.vi"("State(s) in Front (\"\")"="UI: Switch Page >> Settings\nTimer: Stop" ("State(s) in Front (\"\")"), "State(s) in (\"\")"=w336) -> ("States Out"=w335:string)  [unwired: 13 in]
      }
      frame "Macro: Enter Normal Mode" {
        n118 = call <vilib>:"Add State(s) to Queue__JKI_lib_State_Machine.vi"("State(s) in Front (\"\")"="UI: Switch Page >> Normal\nFind Symbol\nCheck If The Symbol Version Exist" ("State(s) in Front (\"\")"), "State(s) in (\"\")"=w342) -> ("States Out"=w341:string)  [unwired: 13 in]
      }
      frame "---------- State Machine ----------" {
        n119 = call <vilib>:"Add State(s) to Queue__JKI_lib_State_Machine.vi"("State(s) in (\"\")"=w347) -> ("States Out"=w346:string)  [unwired: 14 in]
      }
      frame "Excute CMD" {
        n120 = Unbundle By Name(w354) -> ("CMD line"=w348:string)
        n121 = Empty String/Path?(string/path=w348) -> (empty?=w349:bool)
        n122 = case shown="False" w349 {
          tunnel: w348 -> [w357 _]
          tunnel: w351 -> [w356 w360]
          tunnel: [w355 w360] -> w350
          frame False {
            n123 = call <vilib>:"System Exec.vi"("run minimized? (F)"=TRUE, "wait until completion? (T)"=FALSE, "error in (no error)"=w356, "command line"=w357) -> ("error out"=w355:errorcluster)  [unwired: 4 in, 3 out]
          }
          frame True {
          }
        }
      }
      frame "---------- Timer ----------" {
        n124 = call <vilib>:"Add State(s) to Queue__JKI_lib_State_Machine.vi"("State(s) in (\"\")"=w365) -> ("States Out"=w364:string)  [unwired: 14 in]
      }
      frame "Timer: Start" {
        n125 = Get Date/Time In Seconds() -> (seconds since 1Jan1904=w367:timestamp)
        n126 = Bundle By Name(cluster=w369, "Started?"=TRUE ("Timer Info.Started?"), "Start Time"=w367) -> (w368:refnum<class "application.lvclass">)
        n127 = call <vilib>:"Add State(s) to Queue__JKI_lib_State_Machine.vi"("State(s) in (\"\")"=w373) -> ("States Out"=w372:string)  [unwired: 14 in]
      }
      frame "Timer: Stop" {
        n128 = Bundle By Name(cluster=w376, "Started?"=FALSE ("Timer Info.Started?")) -> (w375:refnum<class "application.lvclass">)
        n129 = call <vilib>:"Add State(s) to Queue__JKI_lib_State_Machine.vi"("State(s) in (\"\")"=w380) -> ("States Out"=w379:string)  [unwired: 14 in]
      }
      frame "Timer: Check" {
        n130 = Unbundle By Name(w395) -> ("Started?"=w388:bool, "Start Time"=w394:timestamp, "Display Time(ms)"=w390:i32)
        n131 = Get Date/Time In Seconds() -> (seconds since 1Jan1904=w396:timestamp)
        n132 = To Double Precision Float(number=w396) -> (double precision float=w392:dbl)
        n133 = To Double Precision Float(number=w394) -> (double precision float=w393:dbl)
        n134 = Subtract(x=w392, y=w393) -> (x-y=w391:dbl)
        n135 = To Double Precision Float(number=w390) -> (double precision float=w382:dbl)
        n136 = Divide(x=w382, y=1000.0) -> (x/y=w383:dbl)
        n137 = Greater Or Equal?(x=w391, y=w383) -> (x >= y?=w389:bool)
        n138 = And(x=w388, y=w389) -> (x .and. y?=w387:bool)
        n139 = Select(t="Timer: Timeup", s=w387, f="") -> (s? t:f=w384:string)
        n140 = call <vilib>:"Add State(s) to Queue__JKI_lib_State_Machine.vi"("State(s) in Front (\"\")"=w384, "State(s) in (\"\")"=w400) -> ("States Out"=w399:string)  [unwired: 13 in]
      }
      frame "Timer: Timeup" {
        n141 = call <vilib>:"Add State(s) to Queue__JKI_lib_State_Machine.vi"("State(s) in Front (\"\")"="Macro: OK" ("State(s) in Front (\"\")"), "State(s) in (\"\")"=w406) -> ("States Out"=w405:string)  [unwired: 13 in]
      }
      frame "---------- Actions ----------" {
        n142 = call <vilib>:"Add State(s) to Queue__JKI_lib_State_Machine.vi"("State(s) in (\"\")"=w411) -> ("States Out"=w410:string)  [unwired: 14 in]
      }
      frame "Get Opened File Name" {
        n143 = Unbundle By Name(w416) -> ("RuntimeEngine"=w417:bool)
        n144 = case shown="True" w417 {
          tunnel: w423 -> [w425 w433]
          tunnel: [w425 w432] -> w422
          tunnel: ["file path" w431] -> w418
          tunnel: [FALSE w430] -> w415
          frame False {
          }
          frame True {
            n145 = property class="App"(error in=w433) -> (error out=w432:errorcluster, "App.Args"=w429:string[])  [unwired: 1 in, 1 out]
            n146 = Index Array(array=w429) -> (element #2=w428:string)  [unwired: 2 in, 1 out]
            n147 = String To Path(string=w428) -> (path=w431:path)
            n148 = Empty String/Path?(string/path=w431) -> (empty?=w430:bool)
          }
        }
        n149 = Bundle By Name(cluster=w424, "File Path"=w418) -> (w419:refnum<class "application.lvclass">)
        n150 = Select(t="Macro: Enter Setting Mode", s=w415, f="Macro: Enter Normal Mode") -> (s? t:f=w412:string)
        n151 = call <vilib>:"Add State(s) to Queue__JKI_lib_State_Machine.vi"("State(s) in Front (\"\")"=w412, "State(s) in (\"\")"=w420) -> ("States Out"=w421:string)  [unwired: 13 in]
      }
      frame "Find Symbol" {
        n152 = call <vilib>:"Add State(s) to Queue__JKI_lib_State_Machine.vi"("State(s) in Front (\"\")"="Find New Symbol" ("State(s) at Back (\"\")"), "State(s) in (\"\")"=w437) -> ("States Out"=w438:string)  [unwired: 13 in]
      }
      frame "Find New Symbol" {
        n153 = Unbundle By Name(w450) -> ("File Path"=w453:path)
        n154 = Strip Path(path=w453) -> (stripped path=w441:path)  [unwired: 1 out]
        n155 = call "FindSymbol.vi"("error in (no error)"=w448, "pattern"="DEV ENVIRONMENT *" ("prefix"), "path"=w441) -> ("error out"=w447:errorcluster, "Version"=w452:string, "Exits?"=w440:bool, "Symbol path"=w442:path)  [unwired: 4 in, 1 out]
        n156 = Select(t=w442, s=w440, f=w441) -> (s? t:f=w443:path)
        n157 = Bundle By Name(cluster=w450, "Symbol Path"=w443, "Symbol Version"=w452, "Symbol Found?"=w440) -> (w449:refnum<class "application.lvclass">)
        n158 = Select(t="", s=w440, f="Find Old Symbol" ("State(s) at Back (\"\")")) -> (s? t:f=w444:string)
        n159 = call <vilib>:"Add State(s) to Queue__JKI_lib_State_Machine.vi"("State(s) in Front (\"\")"=w444, "State(s) in (\"\")"=w454) -> ("States Out"=w455:string)  [unwired: 13 in]
      }
      frame "Find Old Symbol" {
        # "If old symbol is found, replace with new symbol."
        n160 = Unbundle By Name(w467) -> ("File Path"=w470:path)
        n161 = Strip Path(path=w470) -> (stripped path=w460:path)  [unwired: 1 out]
        n162 = call "FindSymbol.vi"("error in (no error)"=w465, "pattern"="开发环境 *" ("prefix"), "path"=w460) -> ("error out"=w464:errorcluster, "Version"=w469:string, "Exits?"=w457:bool, "Symbol path"=w458:path)  [unwired: 4 in, 1 out]
        n163 = Select(t=w458, s=w457, f=w460) -> (s? t:f=w459:path)
        n164 = Bundle By Name(cluster=w467, "Symbol Path"=w459, "Symbol Version"=w469, "Symbol Found?"=w457) -> (w466:refnum<class "application.lvclass">)
        n165 = Select(t="Replace with New Symbol", s=w457, f="" ("State(s) at Back (\"\")")) -> (s? t:f=w461:string)
        n166 = call <vilib>:"Add State(s) to Queue__JKI_lib_State_Machine.vi"("State(s) in Front (\"\")"=w461, "State(s) in (\"\")"=w471) -> ("States Out"=w472:string)  [unwired: 13 in]
      }
      frame "Replace with New Symbol" {
        n167 = Unbundle By Name(w476) -> ("Symbol Version"=w478:string, "Symbol Path"=w482:path)
        n168 = call "DeleteSymbolsInDir.vi"("error in (no error)"=w475, "pattern"="开发环境 *", "dup path"=w482) -> ("error in (no error) (dup)"=w480:errorcluster, "dup path (dup)"=w479:path)  [unwired: 7 in]
        n169 = call "CreateSymbolInDir.vi"("error in"=w480, "prefix"="DEV ENVIRONMENT", "Name"=w478, "Path"=w479) -> ("error out"=w474:errorcluster)  [unwired: 6 in, 1 out]
        n170 = call <vilib>:"Add State(s) to Queue__JKI_lib_State_Machine.vi"("State(s) in (\"\")"=w483) -> ("States Out"=w484:string)  [unwired: 14 in]
      }
      frame "Update Symbol" {
        n171 = Unbundle By Name(w490) -> ("Symbol Version"=w488:string, "Selected Version"=w487:string, "Symbol Path"=w489:path)
        n172 = Not Equal?(x=w488, y=w487) -> (x != y?=w486:bool)
        n173 = case shown="True" w486 {
          tunnel: w492 -> [w496 w497]
          tunnel: [w496 w504] -> w491
          tunnel: w489 -> [_ w501]
          tunnel: w487 -> [_ w503]
          frame False {
          }
          frame True {
            n174 = call "DeleteSymbolsInDir.vi"("error in (no error)"=w497, "pattern"="DEV ENVIRONMENT*" ("prefix"), "dup path"=w501) -> ("error in (no error) (dup)"=w498:errorcluster, "dup path (dup)"=w500:path)  [unwired: 7 in]
            n175 = call "CreateSymbolInDir.vi"("error in"=w498, "prefix"="DEV ENVIRONMENT", "Name"=w503, "Path"=w500) -> ("error out"=w504:errorcluster)  [unwired: 6 in, 1 out]
          }
        }
        n176 = call <vilib>:"Add State(s) to Queue__JKI_lib_State_Machine.vi"("State(s) in (\"\")"=w493) -> ("States Out"=w494:string)  [unwired: 14 in]
      }
      frame "Check If The Symbol Version Exist" {
        n177 = Unbundle By Name(w507) -> ("Symbol Found?"=w510:bool, "Version List"=w508:string[], "Symbol Version"=w509:string)
        n178 = case shown="True" w510 {
          tunnel: w508 -> [_ w522]
          tunnel: w509 -> [_ w517]
          tunnel: w507 -> [w515 w520]
          tunnel: [w515 w519] -> w506
          tunnel: [_ w518] -> w505
          frame False {
          }
          frame True {
            n179 = Search 1D Array(1D array=w522, element=w517) -> (index of element=w523:i32)  [unwired: 1 in]
            n180 = Less Than 0?(x=w523) -> (x < 0?=w521:bool)
            n181 = case shown="True" w521 {
              tunnel: ["Timer: Start" _] -> w518
              tunnel: w517 -> [w524 w527]
              tunnel: [w524 w528] -> w516
              frame False {
              }
              frame True {
                n182 = Concatenate Strings(w527, " - Not Exist" ("string")) -> (w528:string)
                n183 = Format Into String(format string="The Symbol Version \"%s\" does not exist on this computer." ("message"), w527) -> (resulting string=w529:string)  [unwired: 2 in, 1 out]
                n184 = One Button Dialog(message=w529) -> ()  [unwired: 1 in, 1 out]
              }
            }
            n185 = Bundle By Name(cluster=w520, "Selected Version"=w516) -> (w519:refnum<class "application.lvclass">)
          }
        }
        n186 = call <vilib>:"Add State(s) to Queue__JKI_lib_State_Machine.vi"("State(s) in Front (\"\")"=w505, "State(s) in (\"\")"=w512) -> ("States Out"=w513:string)  [unwired: 13 in]
      }
      frame "Register Exts" {
        # "#NOTE\ngenerate the Registey Patch file during installation."
        n187 = Merge Errors(w533) -> (w532:errorcluster)
      }
    }
  }
